vi "Configure Output Mode (Pulse-Sweep).vi"(0 "VISA resource name":refnum<visa-resource-name>, 1 "Bias Value (0.0)":dbl min=-15.0 max=15.0 step=1e-07 format="%_5g", 2 "Sweep Range (0: Auto)":u16(ring) items=["Auto", "Fixed"], 5 "Sweep Type  (0: Linear)":i32(ring) items=["Linear", "Fixed Level", "Random", "Two Slope Linear"], 7 "Iteration Count (1)":u16=1 max=1000 step=1, 9 "Enable Reverse Sweep (F: Disable)":bool, 11 "error in (no error)":errorcluster, 12 "Base Value (0.0)":dbl min=-15.0 max=15.0 step=1e-07 format="%_5g", 13 "Enable Return to Bias (T: Enable)":bool=TRUE) -> (4 "VISA resource name out":refnum<visa-resource-name>, 15 "error out":errorcluster)   [LabVIEW 2017, in "ADCMT 6240.lvlib"]
doc: "This VI configure Pulse-Sweep common settings on the instrument.\n<B>Configure Sweep Type VI</B> is used in order to perform a setup for each sweep type."
uses:
  ADCMT 6240.lvlib
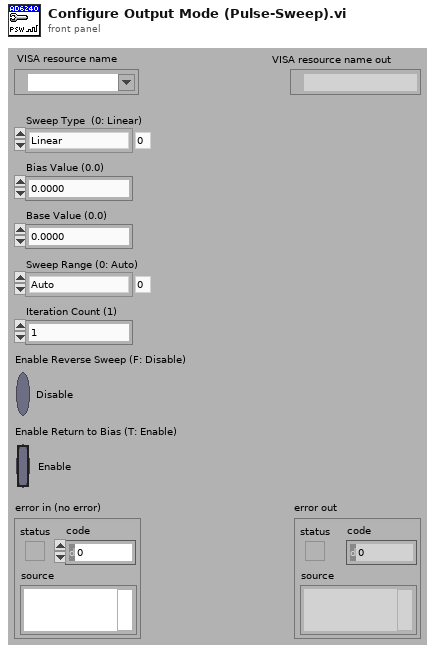
[diagram p1: front panel]
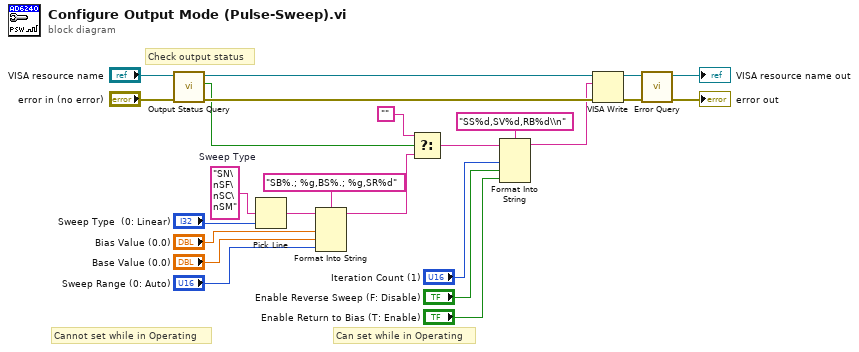
[diagram p0: block diagram]
diagram:
  w13 = "SN\nSF\nSC\nSM"  # Sweep Type
  # "Cannot set while in Operating"
  # "Can set while in Operating"
  # "Check output status"
  n1 = call "Output Status Query.vi"("error in (no error)"="error in (no error)", "VISA resource name"="VISA resource name") -> ("error out"=w16:errorcluster, "Operating"=w10:bool, "VISA resource name out"=w15:refnum<visa-resource-name>)  [unwired: 5 in, 2 out]
  n2 = Pick Line(multi-line string=w13, line index="Sweep Type  (0: Linear)") -> (output string=w11:string)  [unwired: 1 in]
  n3 = Format Into String(format string="SB%.; %g,BS%.; %g,SR%d", initial string=w11, "Bias Value (0.0)", "Base Value (0.0)", "Sweep Range (0: Auto)") -> (resulting string=w8:string)  [unwired: 1 in, 1 out]
  n4 = Select(t="", s=w10, f=w8) -> (s? t:f=w2:string)
  n5 = Format Into String(format string="SS%d,SV%d,RB%d\\n", initial string=w2, "Iteration Count (1)", "Enable Reverse Sweep (F: Disable)", "Enable Return to Bias (T: Enable)") -> (resulting string=w1:string)  [unwired: 1 in, 1 out]
  n6 = VISA Write(VISA resource name=w15, write buffer=w1, error in (no error)=w16) -> (VISA resource name out=w22:refnum<visa-resource-name>, error out=w21:errorcluster)  [unwired: 1 out]
  n7 = call "Error Query.vi"("error in (no error)"=w21, "VISA resource name"=w22) -> ("error out"=→"error out":errorcluster, "VISA resource name out"=→"VISA resource name out":refnum<visa-resource-name>)  [unwired: 6 in, 2 out]
